vi "Lunch menu sub vi.vi"() -> ()   [LabVIEW 2019]
panel:
  out "Desert":string
  out "VEGETABLES":string
  out "Create Your own":string
  out "GRILLED SANDWICH":string
  out "LUNCH ENTREE":string
  out "POTATO & RICE ACCOMPANIMENTS":string
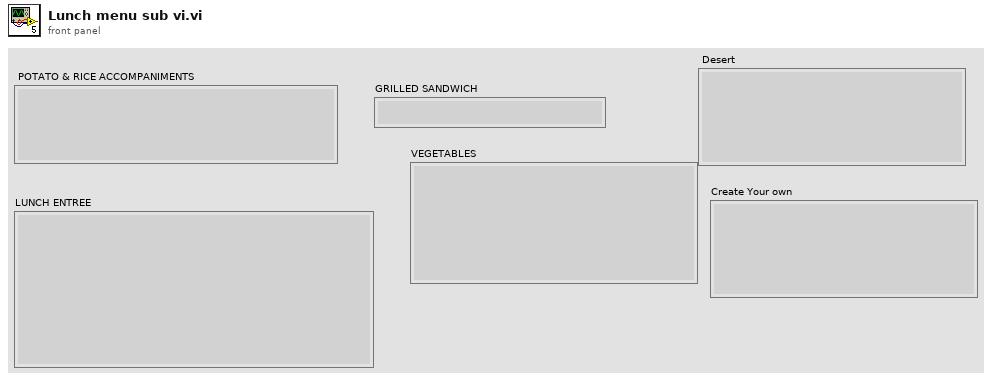
[diagram p1: front panel]
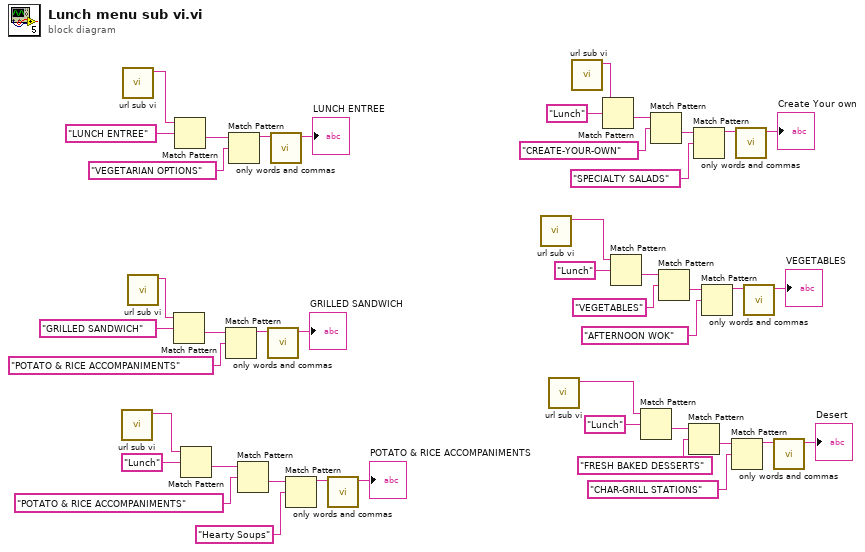
[diagram p0: block diagram]
diagram:
  n1 = call "url sub vi.vi"() -> ("body 2"=w4:string)  [unwired: 11 in]
  n2 = call "url sub vi.vi"() -> ("body 2"=w6:string)  [unwired: 11 in]
  n3 = call "url sub vi.vi"() -> ("body 2"=w5:string)  [unwired: 11 in]
  n4 = Match Pattern(string=w5, regular expression="GRILLED SANDWICH") -> (after substring=w39:string)  [unwired: 1 in, 3 out]
  n5 = Match Pattern(string=w6, regular expression="LUNCH ENTREE") -> (after substring=w43:string)  [unwired: 1 in, 3 out]
  n6 = Match Pattern(string=w4, regular expression="Lunch") -> (after substring=w22:string)  [unwired: 1 in, 3 out]
  n7 = Match Pattern(string=w39, regular expression="POTATO & RICE ACCOMPANIMENTS") -> (before substring=w38:string)  [unwired: 1 in, 3 out]
  n8 = Match Pattern(string=w43, regular expression="VEGETARIAN OPTIONS") -> (before substring=w42:string)  [unwired: 1 in, 3 out]
  n9 = Match Pattern(string=w22, regular expression="POTATO & RICE ACCOMPANIMENTS") -> (after substring=w35:string)  [unwired: 1 in, 3 out]
  n10 = call "only words and commas.vi"("input string"=w38) -> ("result string"=→"GRILLED SANDWICH":string)  [unwired: 10 in]
  n11 = call "only words and commas.vi"("input string"=w42) -> ("result string"=→"LUNCH ENTREE":string)  [unwired: 10 in]
  n12 = Match Pattern(string=w35, regular expression="Hearty Soups") -> (before substring=w25:string)  [unwired: 1 in, 3 out]
  n13 = call "only words and commas.vi"("input string"=w25) -> ("result string"=→"POTATO & RICE ACCOMPANIMENTS":string)  [unwired: 10 in]
  n14 = call "url sub vi.vi"() -> ("body 2"=w2:string)  [unwired: 11 in]
  n15 = call "url sub vi.vi"() -> ("body 2"=w1:string)  [unwired: 11 in]
  n16 = call "url sub vi.vi"() -> ("body 2"=w3:string)  [unwired: 11 in]
  n17 = Match Pattern(string=w3, regular expression="Lunch") -> (after substring=w23:string)  [unwired: 1 in, 3 out]
  n18 = Match Pattern(string=w2, regular expression="Lunch") -> (after substring=w14:string)  [unwired: 1 in, 3 out]
  n19 = Match Pattern(string=w1, regular expression="Lunch") -> (after substring=w7:string)  [unwired: 1 in, 3 out]
  n20 = Match Pattern(string=w23, regular expression="CREATE-YOUR-OWN") -> (after substring=w32:string)  [unwired: 1 in, 3 out]
  n21 = Match Pattern(string=w14, regular expression="VEGETABLES") -> (after substring=w19:string)  [unwired: 1 in, 3 out]
  n22 = Match Pattern(string=w7, regular expression="FRESH BAKED DESSERTS") -> (after substring=w12:string)  [unwired: 1 in, 3 out]
  n23 = Match Pattern(string=w32, regular expression="SPECIALTY SALADS") -> (before substring=w31:string)  [unwired: 1 in, 3 out]
  n24 = Match Pattern(string=w19, regular expression="AFTERNOON WOK") -> (before substring=w18:string)  [unwired: 1 in, 3 out]
  n25 = Match Pattern(string=w12, regular expression="CHAR-GRILL STATIONS") -> (before substring=w11:string)  [unwired: 1 in, 3 out]
  n26 = call "only words and commas.vi"("input string"=w31) -> ("result string"=→"Create Your own":string)  [unwired: 10 in]
  n27 = call "only words and commas.vi"("input string"=w18) -> ("result string"=→"VEGETABLES":string)  [unwired: 10 in]
  n28 = call "only words and commas.vi"("input string"=w11) -> ("result string"=→"Desert":string)  [unwired: 10 in]
